vi "Charger_Is Charge Done.vi"(7 "Status Refnum":T1, 8 "error in":errorcluster) -> (0 "error out":errorcluster, 4 "done":bool)   [LabVIEW 2020]
uses:
  Charger_Status Refnum.ctl
  Drivers/Charger Test Set/Charger_Input Control.ctl
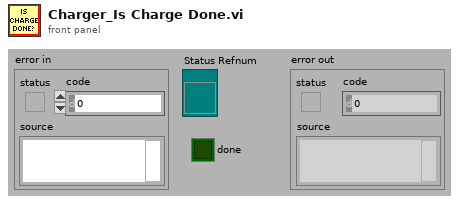
[diagram p1: front panel]
types:
  T1 = typedef "Charger_Status Refnum.ctl" = refnum<vi>
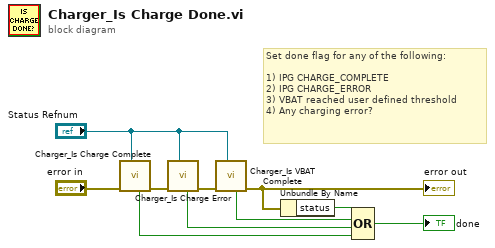
[diagram p0: block diagram]
diagram:
  # "Set done flag for any of the following:\n\n1) IPG CHARGE_COMPLETE\n2) IPG CHARGE_ERROR\n3) VBAT reached user defined threshold\n4) Any charging error?"
  n1 = call "Charger_Is Charge Complete.vi"("Status Refnum"="Status Refnum", "error in"="error in") -> ("error out"=w10:errorcluster, "complete"=w8:bool)  [unwired: 8 in]
  n2 = call "Charger_Is Charge Error.vi"("Status Refnum"="Status Refnum", "error in"=w10) -> ("error out"=w5:errorcluster, "complete"=w1:bool)  [unwired: 8 in]
  n3 = call "Charger_Is VBAT Complete.vi"("Status Refnum"="Status Refnum", "error in"=w5) -> ("error out"=w4:errorcluster, "complete"=w2:bool)  [unwired: 8 in]
  "error out" <- w4
  n4 = Unbundle By Name(w4) -> ("status"=w7:bool)
  n5 = Compound Arithmetic op=OR(w7, w2, w1, w8) -> (→"done":bool)
